vi "InitialiseOLED.vi"(8 "error in (no error)":errorcluster) -> (0 "error out":errorcluster, 3 "Messages":string[](array[string]))   [LabVIEW 2020, in "CTI-Peripheral.lvlib" / "64x128 I2C OLED SSD1315.lvclass"]
uses:
  64x128 I2C OLED SSD1315.lvclass
  Command.ctl
  Address Mode.ctl
  64x128 I2C OLED SSD1315.lvclass/64x128 I2C OLED SSD1315.ctl
panel:
  # "Input"
  # "Output"
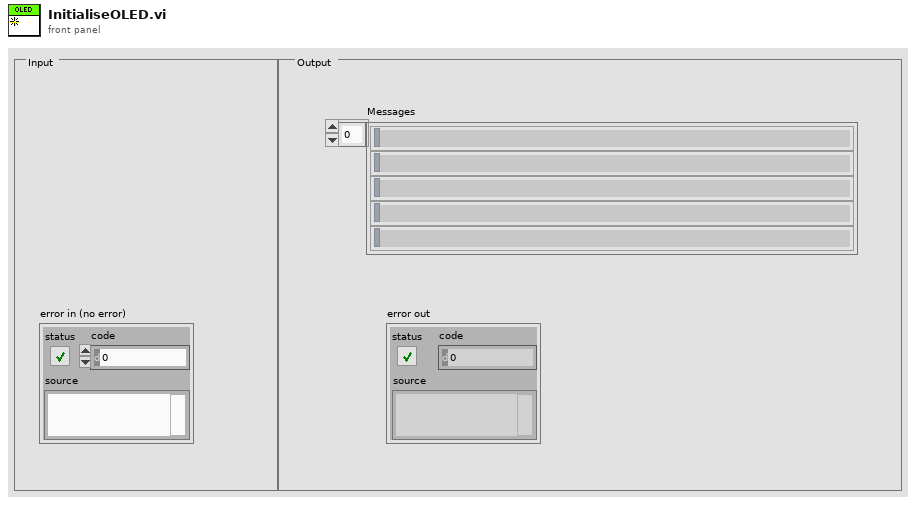
[diagram p1: front panel]
types:
  T1 = typedef "CTI-Peripheral.lvlib/64x128 I2C OLED SSD1315.lvclass/Command.ctl" = u8
  T2 = typedef "CTI-Peripheral.lvlib/64x128 I2C OLED SSD1315.lvclass/Address Mode.ctl" = enum16{"Horizontal", "Vertical", "Page"}
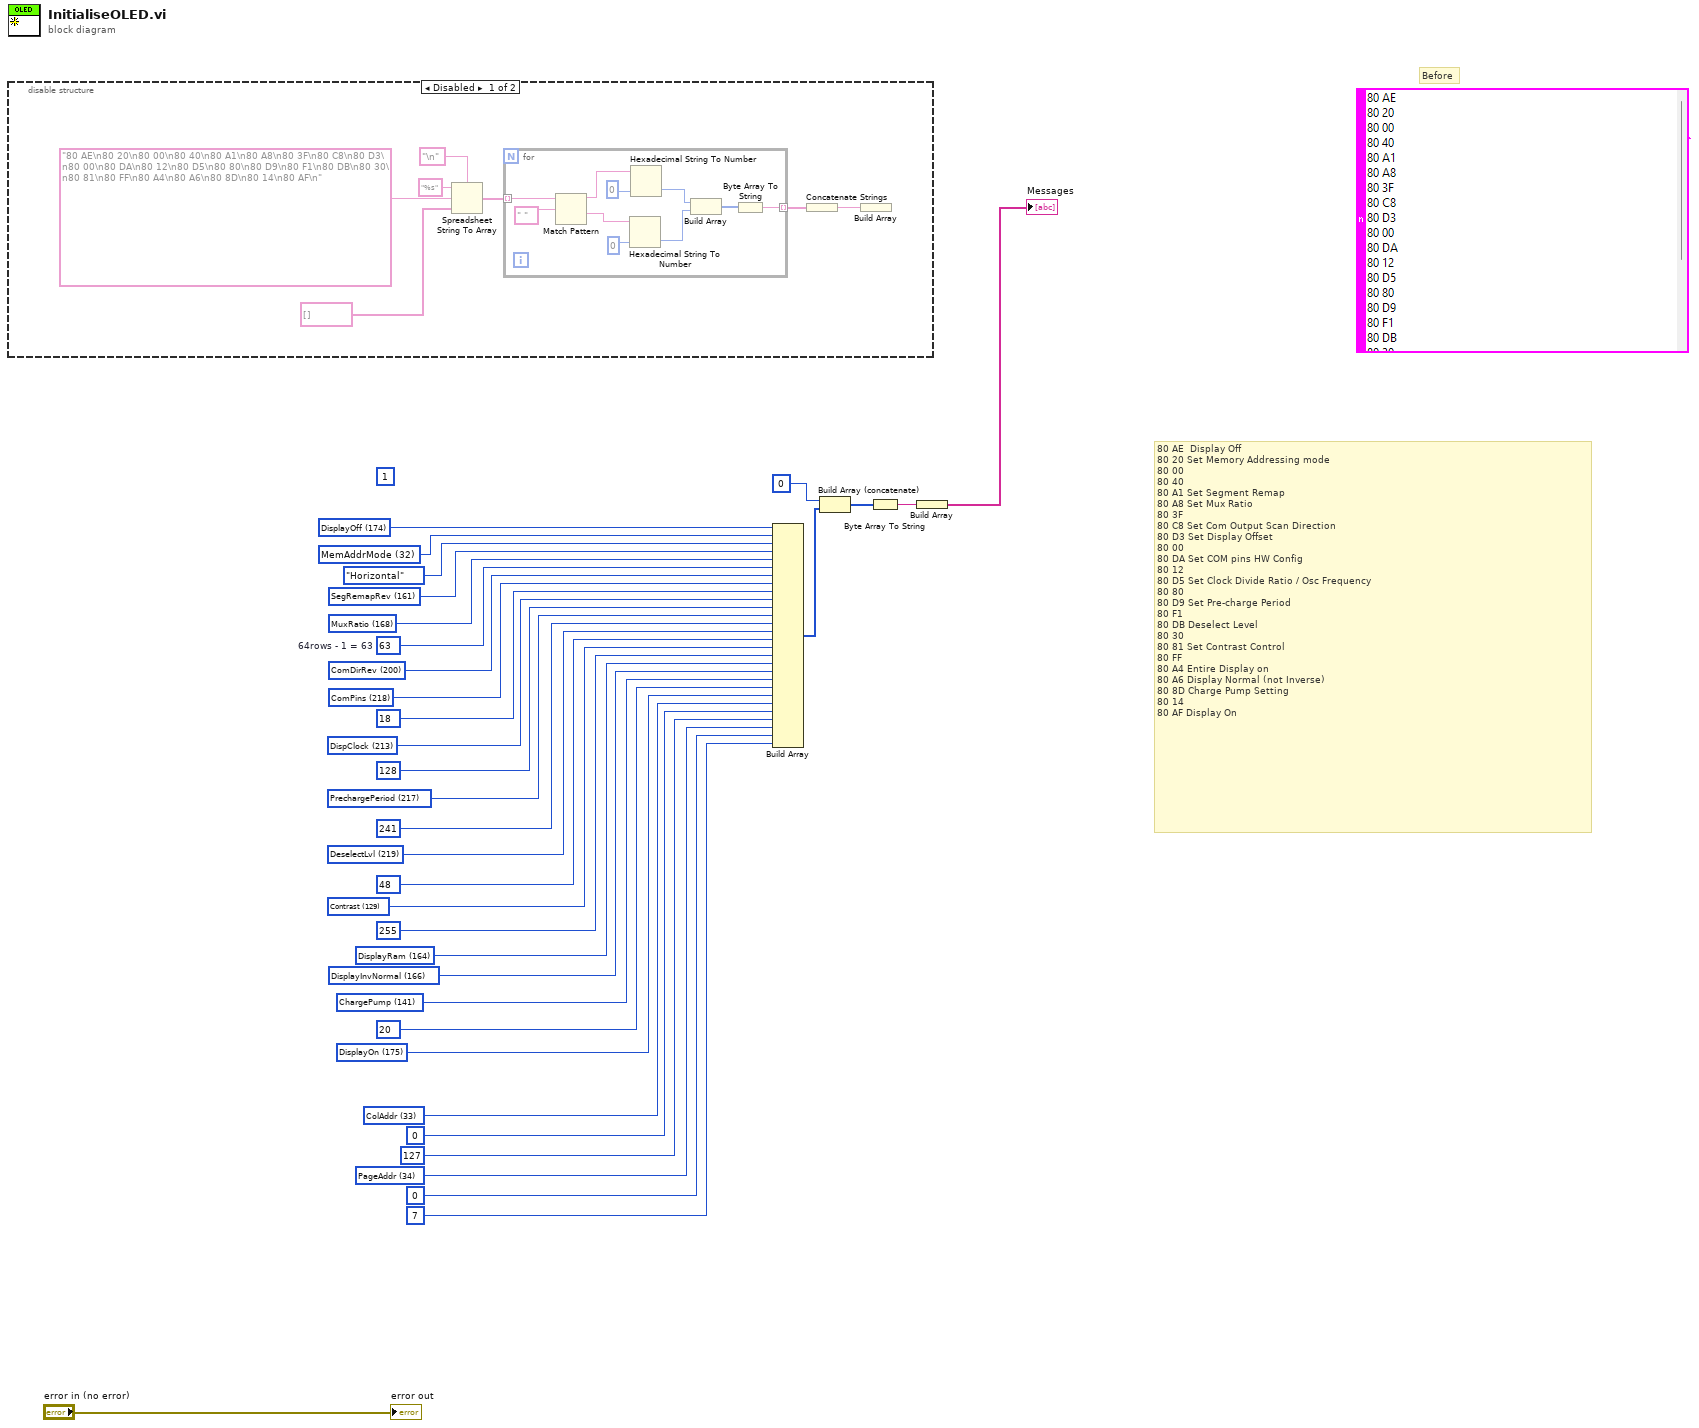
[diagram p0: block diagram]
diagram:
  w3 = T1 34 items=["StartColLow"=0, "StartColHigh"=16, "MemAddrMode"=32, "ColAddr"=33, "PageAddr"=34, "ScrollH"=38, "ScrollVH"=41, "ScrollOff"=46, "ScrollOn"=47, "StartLine"=64, "Contrast"=129, "ChargePump"=141, "SegRemapFwd"=160, "SegRemapRev"=161, "ScrollVArea"=163, "DisplayRam"=164, "DisplayAllOn"=165, "DisplayInvNormal"=166, "DisplayInverted"=167, "MuxRatio"=168, "DisplayOff"=174, "DisplayOn"=175, "PageStart"=176, "ComDirFwd"=192, "ComDirRev"=200, "DispOffset"=211, "DispClock"=213, "PrechargePeriod"=217, "ComPins"=218, "DeselectLvl"=219, "Noop"=227] ("Command")
  w6 = T1 33 items=["StartColLow"=0, "StartColHigh"=16, "MemAddrMode"=32, "ColAddr"=33, "PageAddr"=34, "ScrollH"=38, "ScrollVH"=41, "ScrollOff"=46, "ScrollOn"=47, "StartLine"=64, "Contrast"=129, "ChargePump"=141, "SegRemapFwd"=160, "SegRemapRev"=161, "ScrollVArea"=163, "DisplayRam"=164, "DisplayAllOn"=165, "DisplayInvNormal"=166, "DisplayInverted"=167, "MuxRatio"=168, "DisplayOff"=174, "DisplayOn"=175, "PageStart"=176, "ComDirFwd"=192, "ComDirRev"=200, "DispOffset"=211, "DispClock"=213, "PrechargePeriod"=217, "ComPins"=218, "DeselectLvl"=219, "Noop"=227] ("Command")
  w8 = T1 175 items=["StartColLow"=0, "StartColHigh"=16, "MemAddrMode"=32, "ColAddr"=33, "PageAddr"=34, "ScrollH"=38, "ScrollVH"=41, "ScrollOff"=46, "ScrollOn"=47, "StartLine"=64, "Contrast"=129, "ChargePump"=141, "SegRemapFwd"=160, "SegRemapRev"=161, "ScrollVArea"=163, "DisplayRam"=164, "DisplayAllOn"=165, "DisplayInvNormal"=166, "DisplayInverted"=167, "MuxRatio"=168, "DisplayOff"=174, "DisplayOn"=175, "PageStart"=176, "ComDirFwd"=192, "ComDirRev"=200, "DispOffset"=211, "DispClock"=213, "PrechargePeriod"=217, "ComPins"=218, "DeselectLvl"=219, "Noop"=227] ("Command")
  w10 = T1 141 items=["StartColLow"=0, "StartColHigh"=16, "MemAddrMode"=32, "ColAddr"=33, "PageAddr"=34, "ScrollH"=38, "ScrollVH"=41, "ScrollOff"=46, "ScrollOn"=47, "StartLine"=64, "Contrast"=129, "ChargePump"=141, "SegRemapFwd"=160, "SegRemapRev"=161, "ScrollVArea"=163, "DisplayRam"=164, "DisplayAllOn"=165, "DisplayInvNormal"=166, "DisplayInverted"=167, "MuxRatio"=168, "DisplayOff"=174, "DisplayOn"=175, "PageStart"=176, "ComDirFwd"=192, "ComDirRev"=200, "DispOffset"=211, "DispClock"=213, "PrechargePeriod"=217, "ComPins"=218, "DeselectLvl"=219, "Noop"=227] ("Command")
  w14 = T1 129 items=["StartColLow"=0, "StartColHigh"=16, "MemAddrMode"=32, "ColAddr"=33, "PageAddr"=34, "ScrollH"=38, "ScrollVH"=41, "ScrollOff"=46, "ScrollOn"=47, "StartLine"=64, "Contrast"=129, "SegRemapFwd"=160, "SegRemapRev"=161, "ScrollVArea"=163, "DisplayRam"=164, "DisplayAllOn"=165, "DisplayInvNormal"=166, "DisplayInverted"=167, "MuxRatio"=168, "DisplayOff"=174, "DisplayOn"=175, "PageStart"=176, "ComDirFwd"=192, "ComDirRev"=200, "DispOffset"=211, "DispClock"=213, "PrechargePeriod"=217, "ComPins"=218, "DeselectLvl"=219, "Noop"=227] ("Command")
  w16 = T1 219 items=["StartColLow"=0, "StartColHigh"=16, "MemAddrMode"=32, "ColAddr"=33, "PageAddr"=34, "ScrollH"=38, "ScrollVH"=41, "ScrollOff"=46, "ScrollOn"=47, "StartLine"=64, "Contrast"=129, "SegRemapFwd"=160, "SegRemapRev"=161, "ScrollVArea"=163, "DisplayRam"=164, "DisplayAllOn"=165, "DisplayInvNormal"=166, "DisplayInverted"=167, "MuxRatio"=168, "DisplayOff"=174, "DisplayOn"=175, "PageStart"=176, "ComDirFwd"=192, "ComDirRev"=200, "DispOffset"=211, "DispClock"=213, "PrechargePeriod"=217, "ComPins"=218, "DeselectLvl"=219, "Noop"=227] ("Command")
  w18 = T1 217 items=["StartColLow"=0, "StartColHigh"=16, "MemAddrMode"=32, "ColAddr"=33, "PageAddr"=34, "ScrollH"=38, "ScrollVH"=41, "ScrollOff"=46, "ScrollOn"=47, "StartLine"=64, "Contrast"=129, "SegRemapFwd"=160, "SegRemapRev"=161, "ScrollVArea"=163, "DisplayRam"=164, "DisplayAllOn"=165, "DisplayInvNormal"=166, "DisplayInverted"=167, "MuxRatio"=168, "DisplayOff"=174, "DisplayOn"=175, "PageStart"=176, "ComDirFwd"=192, "ComDirRev"=200, "DispOffset"=211, "DispClock"=213, "PrechargePeriod"=217, "ComPins"=218, "DeselectLvl"=219, "Noop"=227] ("Command")
  w20 = T1 213 items=["StartColLow"=0, "StartColHigh"=16, "MemAddrMode"=32, "ColAddr"=33, "PageAddr"=34, "ScrollH"=38, "ScrollVH"=41, "ScrollOff"=46, "ScrollOn"=47, "StartLine"=64, "Contrast"=129, "SegRemapFwd"=160, "SegRemapRev"=161, "ScrollVArea"=163, "DisplayRam"=164, "DisplayAllOn"=165, "DisplayInvNormal"=166, "DisplayInverted"=167, "MuxRatio"=168, "DisplayOff"=174, "DisplayOn"=175, "PageStart"=176, "ComDirFwd"=192, "ComDirRev"=200, "DispOffset"=211, "DispClock"=213, "PrechargePeriod"=217, "ComPins"=218, "DeselectLvl"=219, "Noop"=227] ("Command")
  w11 = T1 166 items=["StartColLow"=0, "StartColHigh"=16, "MemAddrMode"=32, "ColAddr"=33, "PageAddr"=34, "ScrollH"=38, "ScrollVH"=41, "ScrollOff"=46, "ScrollOn"=47, "StartLine"=64, "Contrast"=129, "SegRemapFwd"=160, "SegRemapRev"=161, "ScrollVArea"=163, "DisplayRam"=164, "DisplayAllOn"=165, "DisplayInvNormal"=166, "DisplayInverted"=167, "MuxRatio"=168, "DisplayOff"=174, "DisplayOn"=175, "PageStart"=176, "ComDirFwd"=192, "ComDirRev"=200, "DispOffset"=211, "DispClock"=213, "PrechargePeriod"=217, "ComPins"=218, "DeselectLvl"=219, "Noop"=227] ("Command")
  w12 = T1 164 items=["StartColLow"=0, "StartColHigh"=16, "MemAddrMode"=32, "ColAddr"=33, "PageAddr"=34, "ScrollH"=38, "ScrollVH"=41, "ScrollOff"=46, "ScrollOn"=47, "StartLine"=64, "Contrast"=129, "SegRemapFwd"=160, "SegRemapRev"=161, "ScrollVArea"=163, "DisplayRam"=164, "DisplayAllOn"=165, "DisplayInvNormal"=166, "DisplayInverted"=167, "MuxRatio"=168, "DisplayOff"=174, "DisplayOn"=175, "PageStart"=176, "ComDirFwd"=192, "ComDirRev"=200, "DispOffset"=211, "DispClock"=213, "PrechargePeriod"=217, "ComPins"=218, "DeselectLvl"=219, "Noop"=227] ("Command")
  w22 = T1 218 items=["StartColLow"=0, "StartColHigh"=16, "MemAddrMode"=32, "ColAddr"=33, "PageAddr"=34, "ScrollH"=38, "ScrollVH"=41, "ScrollOff"=46, "ScrollOn"=47, "StartLine"=64, "Contrast"=129, "SegRemapFwd"=160, "SegRemapRev"=161, "ScrollVArea"=163, "DisplayRam"=164, "DisplayAllOn"=165, "DisplayInvNormal"=166, "DisplayInverted"=167, "MuxRatio"=168, "DisplayOff"=174, "DisplayOn"=175, "PageStart"=176, "ComDirFwd"=192, "ComDirRev"=200, "DispOffset"=211, "DispClock"=213, "PrechargePeriod"=217, "ComPins"=218, "DeselectLvl"=219, "Noop"=227] ("Command")
  w27 = T1 200 items=["StartColLow"=0, "StartColHigh"=16, "MemAddrMode"=32, "ColAddr"=33, "PageAddr"=34, "ScrollH"=38, "ScrollVH"=41, "ScrollOff"=46, "ScrollOn"=47, "StartLine"=64, "Contrast"=129, "SegRemapFwd"=160, "SegRemapRev"=161, "ScrollVArea"=163, "DisplayRam"=164, "DisplayAllOn"=165, "DisplayInvNormal"=166, "DisplayInverted"=167, "MuxRatio"=168, "DisplayOff"=174, "DisplayOn"=175, "PageStart"=176, "ComDirFwd"=192, "ComDirRev"=200, "DispOffset"=211, "DispClock"=213, "PrechargePeriod"=217, "ComPins"=218, "DeselectLvl"=219, "Noop"=227] ("Command")
  w28 = u8 63  # 64rows - 1 = 63
  w29 = T1 168 items=["StartColLow"=0, "StartColHigh"=16, "MemAddrMode"=32, "ColAddr"=33, "PageAddr"=34, "ScrollH"=38, "ScrollVH"=41, "ScrollOff"=46, "ScrollOn"=47, "StartLine"=64, "Contrast"=129, "SegRemapFwd"=160, "SegRemapRev"=161, "ScrollVArea"=163, "DisplayRam"=164, "DisplayAllOn"=165, "DisplayInvNormal"=166, "DisplayInverted"=167, "MuxRatio"=168, "DisplayOff"=174, "DisplayOn"=175, "PageStart"=176, "ComDirFwd"=192, "ComDirRev"=200, "DispOffset"=211, "DispClock"=213, "PrechargePeriod"=217, "ComPins"=218, "DeselectLvl"=219, "Noop"=227] ("Command")
  w30 = T1 161 items=["StartColLow"=0, "StartColHigh"=16, "MemAddrMode"=32, "ColAddr"=33, "PageAddr"=34, "ScrollH"=38, "ScrollVH"=41, "ScrollOff"=46, "ScrollOn"=47, "StartLine"=64, "Contrast"=129, "SegRemapFwd"=160, "SegRemapRev"=161, "ScrollVArea"=163, "DisplayRam"=164, "DisplayAllOn"=165, "DisplayInvNormal"=166, "DisplayInverted"=167, "MuxRatio"=168, "DisplayOff"=174, "DisplayOn"=175, "PageStart"=176, "ComDirFwd"=192, "ComDirRev"=200, "DispOffset"=211, "DispClock"=213, "PrechargePeriod"=217, "ComPins"=218, "DeselectLvl"=219, "Noop"=227] ("Command")
  (unwired) u8 1
  w32 = T1 32 items=["StartColLow"=0, "StartColHigh"=16, "MemAddrMode"=32, "ColAddr"=33, "PageAddr"=34, "ScrollH"=38, "ScrollVH"=41, "ScrollOff"=46, "ScrollOn"=47, "StartLine"=64, "Contrast"=129, "SegRemap"=160, "ScrollVArea"=163, "DisplayRam"=164, "DisplayAllOn"=165, "DisplayInvNormal"=166, "DisplayInverted"=167, "MuxRatio"=168, "DisplayOff"=174, "DisplayOn"=175, "PageStart"=176, "ComDirFwd"=192, "ComDirRev"=200, "DispOffset"=211, "DispClock"=213, "PrechargePeriod"=217, "ComPins"=218, "DeselectLvl"=219, "Noop"=227] ("Command")
  w33 = T1 174 items=["StartColLow"=0, "StartColHigh"=16, "MemAddrMode"=32, "ColAddr"=33, "PageAddr"=34, "ScrollH"=38, "ScrollVH"=41, "ScrollOff"=46, "ScrollOn"=47, "StartLine"=64, "Contrast"=129, "SegRemap"=160, "ScrollVArea"=163, "DisplayRam"=164, "DisplayAllOn"=165, "DisplayInvNormal"=166, "DisplayInverted"=167, "MuxRatio"=168, "DisplayOff"=174, "DisplayOn"=175, "PageStart"=176, "ComDirFwd"=192, "ComDirRev"=200, "DispOffset"=211, "DispClock"=213, "PrechargePeriod"=217, "ComPins"=218, "DeselectLvl"=219, "Noop"=227] ("Command")
  # "Before"
  # "80 AE  Display Off\n80 20 Set Memory Addressing mode\n80 00 \n80 40\n80 A1 Set Segment Remap\n80 A8 Set Mux Ratio\n80 3F\n80 C8 Set Com Output Scan Direction\n80 D3 Set Display Offset\n80 00\n80 DA Set COM pins HW Config\n80 12\n80 D5 Set Clock Divide Ratio / Osc Frequency\n80 80\n80 D9 Set Pre-charge Period\n80 F1\n80 DB Deselect Level\n80 30\n80 81 Set Contrast Control\n80 FF\n80 A4 Entire Display on\n80 A6 Display Normal (not Inverse)\n80 8D Charge Pump Setting\n80 14\n80 AF Display On"
  n1 = disable-structure shown="Disabled" {
    frame Disabled {
      n2 = Spreadsheet String To Array(delimiter (Tab)="\n", format string="%s", spreadsheet string="80 AE\n80 20\n80 00\n80 40\n80 A1\n80 A8\n80 3F\n80 C8\n80 D3\n80 00\n80 DA\n80 12\n80 D5\n80 80\n80 D9\n80 F1\n80 DB\n80 30\n80 81\n80 FF\n80 A4\n80 A6\n80 8D\n80 14\n80 AF\n", array type (2D Dbl)=string[] []) -> (array=w37:string[])
      n3 = for {
        tunnel: w37 -> [w48] mode=indexing
        tunnel: [w44] -> w36 mode=indexing
        n4 = Match Pattern(string=w48, regular expression=" " ("delimiter (Tab)")) -> (before substring=w50:string, after substring=w49:string)  [unwired: 1 in, 2 out]
        n5 = Hexadecimal String To Number(string=w49, default (0uL)=u8 0) -> (number=w46:u8)  [unwired: 1 in, 1 out]
        n6 = Hexadecimal String To Number(string=w50, default (0uL)=u8 0) -> (number=w47:u8)  [unwired: 1 in, 1 out]
        n7 = Build Array(w47, w46) -> (w45:u8[])
        n8 = Byte Array To String(unsigned byte array=w45) -> (string=w44:string)
      }
      n9 = Concatenate Strings(w36) -> (w35:string)
      n10 = Build Array(w35) -> ()  [unwired: 1 out]
    }
    frame Enabled {
    }
  }
  n11 = Build Array(w33, w32, Address_Mode."Horizontal" ("Address Mode"), w30, w29, w28, w27, w22, u8 18, w20, u8 128, w18, u8 241, w16, u8 48, w14, u8 255, w12, w11, w10, u8 20, w8, w6, u8 0 ("element"), u8 127 ("element"), w3, u8 0 ("element"), u8 7 ("element")) -> (w26:u16[])
  n12 = Build Array (concatenate)(u8 0, w26) -> (w24:u16[])
  n13 = Byte Array To String(unsigned byte array=w24) -> (string=w23:string)
  n14 = Build Array(w23) -> (→"Messages":string[])
  "error out" <- "error in (no error)"
